vi "UIinit_MergeFile.vi"(10 "Language":u32, 11 "VI输入":refnum<vi>) -> ()   [LabVIEW 2015]
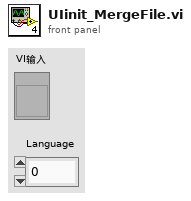
[diagram p1: front panel]
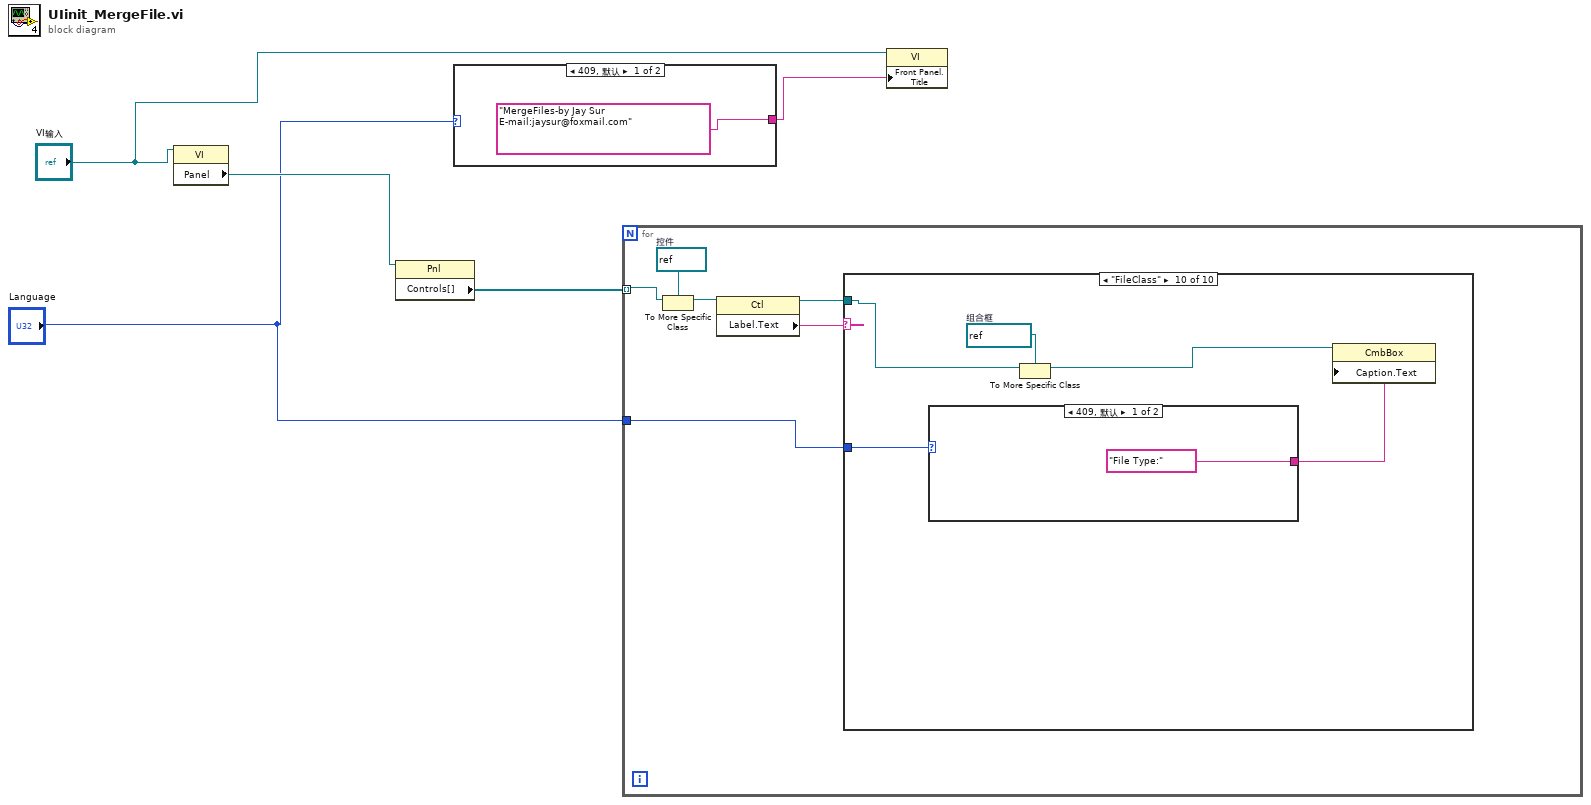
[diagram p0: block diagram]
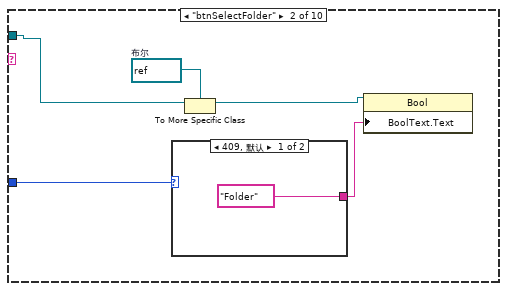
[diagram p3: hidden frame]
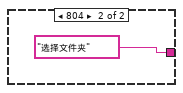
[diagram p4: hidden frame]
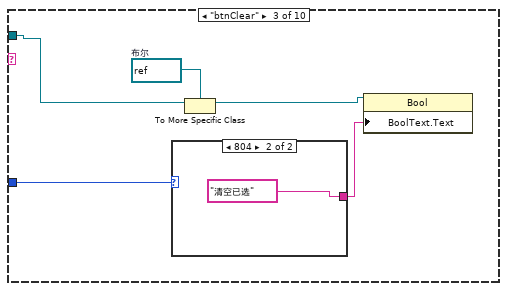
[diagram p5: hidden frame]
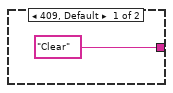
[diagram p6: hidden frame]
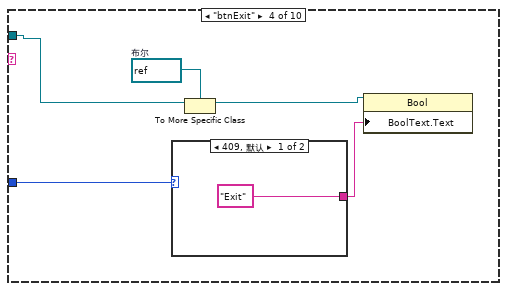
[diagram p7: hidden frame]
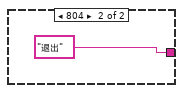
[diagram p8: hidden frame]
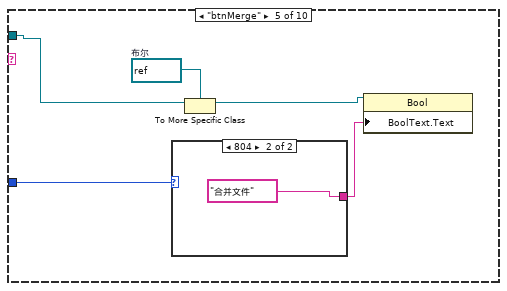
[diagram p9: hidden frame]
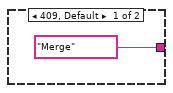
[diagram p10: hidden frame]
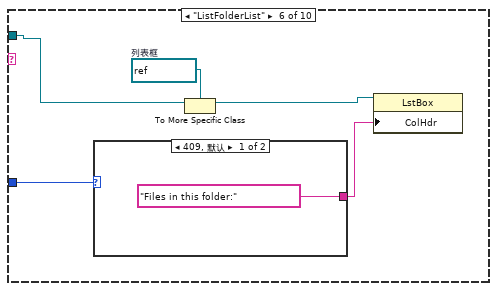
[diagram p11: hidden frame]
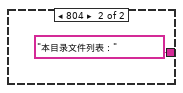
[diagram p12: hidden frame]
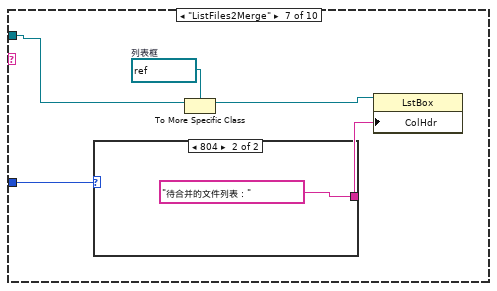
[diagram p13: hidden frame]
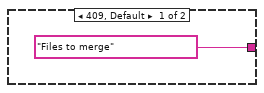
[diagram p14: hidden frame]
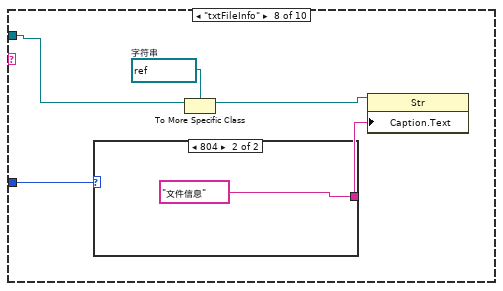
[diagram p15: hidden frame]
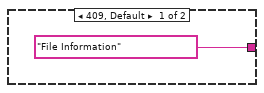
[diagram p16: hidden frame]
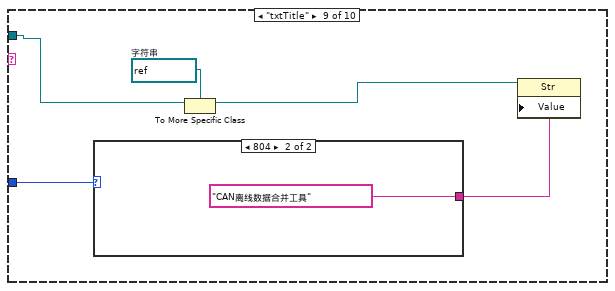
[diagram p17: hidden frame]
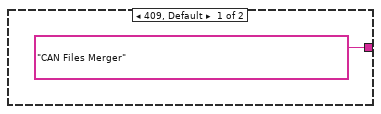
[diagram p18: hidden frame]
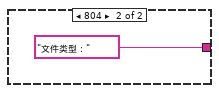
[diagram p19: hidden frame]
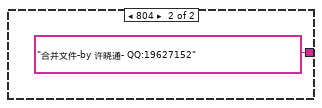
[diagram p20: hidden frame]
diagram:
  n1 = property class="VI"(reference="VI输入") -> ("Panel"=w3:refnum<vi>)  [unwired: 1 in, 2 out]
  n2 = property class="Pnl"(reference=w3) -> ("Controls[]"=w2:refnum<vi>[])  [unwired: 1 in, 2 out]
  n3 = case shown="409, 默认" "Language" {
    tunnel: ["MergeFiles-by Jay Sur E-mail:jaysur@foxmail.com" "合并文件-by 许晓通- QQ:19627152"] -> w5
    frame 409, Default {
    }
    frame 804 {
    }
  }
  n4 = for {
    tunnel: w2 -> [w11] mode=indexing
    tunnel: "Language" -> [w8]
    w13 = refnum<vi> refnum  # 控件
    n5 = To More Specific Class(target class=w13, reference=w11) -> (specific class reference=w12:refnum<vi>)  [unwired: 1 in, 1 out]
    n6 = property class="Ctl"(reference=w12) -> (reference out=w9:refnum<vi>, "Label.Text"=w10:string)  [unwired: 1 in, 1 out]
    n7 = case shown="\"FileClass\"" w10 {
      tunnel: w9 -> [_ w15 w22 w29 w36 w43 w50 w57 w64 w71]
      tunnel: w8 -> [_ w14 w21 w28 w35 w42 w49 w56 w63 w70]
      frame "假", Default {
      }
      frame "btnSelectFolder" {
        w18 = refnum<vi> refnum  # 布尔
        n8 = case shown="409, 默认" w14 {
          tunnel: ["Folder" "选择文件夹"] -> w16
          frame 409, Default {
          }
          frame 804 {
          }
        }
        n9 = To More Specific Class(target class=w18, reference=w15) -> (specific class reference=w17:refnum<vi>)  [unwired: 1 in, 1 out]
        n10 = property class="Bool"(reference=w17, "BoolText.Text"=w16) -> ()  [unwired: 1 in, 2 out]
      }
      frame "btnClear" {
        w25 = refnum<vi> refnum  # 布尔
        n11 = case shown="804" w21 {
          tunnel: ["Clear" "清空已选"] -> w23
          frame 409, Default {
          }
          frame 804 {
          }
        }
        n12 = To More Specific Class(target class=w25, reference=w22) -> (specific class reference=w24:refnum<vi>)  [unwired: 1 in, 1 out]
        n13 = property class="Bool"(reference=w24, "BoolText.Text"=w23) -> ()  [unwired: 1 in, 2 out]
      }
      frame "btnExit" {
        w32 = refnum<vi> refnum  # 布尔
        n14 = case shown="409, 默认" w28 {
          tunnel: ["Exit" "退出"] -> w30
          frame 409, Default {
          }
          frame 804 {
          }
        }
        n15 = To More Specific Class(target class=w32, reference=w29) -> (specific class reference=w31:refnum<vi>)  [unwired: 1 in, 1 out]
        n16 = property class="Bool"(reference=w31, "BoolText.Text"=w30) -> ()  [unwired: 1 in, 2 out]
      }
      frame "btnMerge" {
        w39 = refnum<vi> refnum  # 布尔
        n17 = case shown="804" w35 {
          tunnel: ["Merge" "合并文件"] -> w37
          frame 409, Default {
          }
          frame 804 {
          }
        }
        n18 = To More Specific Class(target class=w39, reference=w36) -> (specific class reference=w38:refnum<vi>)  [unwired: 1 in, 1 out]
        n19 = property class="Bool"(reference=w38, "BoolText.Text"=w37) -> ()  [unwired: 1 in, 2 out]
      }
      frame "ListFolderList" {
        w46 = refnum<vi> refnum  # 列表框
        n20 = case shown="409, 默认" w42 {
          tunnel: ["Files in this folder:" "本目录文件列表："] -> w44
          frame 409, Default {
          }
          frame 804 {
          }
        }
        n21 = To More Specific Class(target class=w46, reference=w43) -> (specific class reference=w45:refnum<vi>)  [unwired: 1 in, 1 out]
        n22 = property class="LstBox"(reference=w45, "ColHdr"=w44) -> ()  [unwired: 1 in, 2 out]
      }
      frame "ListFiles2Merge" {
        w53 = refnum<vi> refnum  # 列表框
        n23 = case shown="804" w49 {
          tunnel: ["Files to merge" "待合并的文件列表："] -> w51
          frame 409, Default {
          }
          frame 804 {
          }
        }
        n24 = To More Specific Class(target class=w53, reference=w50) -> (specific class reference=w52:refnum<vi>)  [unwired: 1 in, 1 out]
        n25 = property class="LstBox"(reference=w52, "ColHdr"=w51) -> ()  [unwired: 1 in, 2 out]
      }
      frame "txtFileInfo" {
        w60 = refnum<vi> refnum  # 字符串
        n26 = case shown="804" w56 {
          tunnel: ["File Information" "文件信息"] -> w58
          frame 409, Default {
          }
          frame 804 {
          }
        }
        n27 = To More Specific Class(target class=w60, reference=w57) -> (specific class reference=w59:refnum<vi>)  [unwired: 1 in, 1 out]
        n28 = property class="Str"(reference=w59, "Caption.Text"=w58) -> ()  [unwired: 1 in, 2 out]
      }
      frame "txtTitle" {
        w67 = refnum<vi> refnum  # 字符串
        n29 = case shown="804" w63 {
          tunnel: ["CAN Files Merger" "CAN离线数据合并工具"] -> w65
          frame 409, Default {
          }
          frame 804 {
          }
        }
        n30 = To More Specific Class(target class=w67, reference=w64) -> (specific class reference=w66:refnum<vi>)  [unwired: 1 in, 1 out]
        n31 = property class="Str"(reference=w66, "Value"=w65) -> ()  [unwired: 1 in, 2 out]
      }
      frame "FileClass" {
        w74 = refnum<vi> refnum  # 组合框
        n32 = case shown="409, 默认" w70 {
          tunnel: ["File Type:" "文件类型："] -> w72
          frame 409, Default {
          }
          frame 804 {
          }
        }
        n33 = To More Specific Class(target class=w74, reference=w71) -> (specific class reference=w73:refnum<vi>)  [unwired: 1 in, 1 out]
        n34 = property class="CmbBox"(reference=w73, "Caption.Text"=w72) -> ()  [unwired: 1 in, 2 out]
      }
    }
  }
  n35 = property class="VI"(reference="VI输入", "Front Panel.Title"=w5) -> ()  [unwired: 1 in, 2 out]
